vi "read_attributes.vi"(8 "error in (no error)":errorcluster, 11 "RadiusNeighborsRegressor in":refnum<class "RadiusNeighborsRegressor.lvclass">) -> (0 "error out":errorcluster, 2 "attributes":T1, 3 "RadiusNeighborsRegressor out":refnum<class "RadiusNeighborsRegressor.lvclass">)   [LabVIEW 2020, in "RadiusNeighborsRegressor.lvclass"]
uses:
  RadiusNeighborsRegressor.lvclass
  Controls/radius_neighbors_regressor_attributes.ctl
  RadiusNeighborsRegressor.lvclass/RadiusNeighborsRegressor.ctl
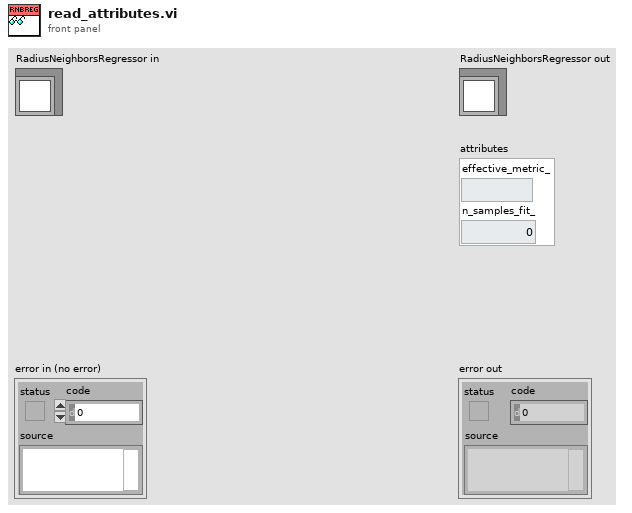
[diagram p1: front panel]
types:
  T1 = typedef "radius_neighbors_regressor_attributes.ctl" = cluster{"effective_metric_":string, "n_samples_fit_":dbl}
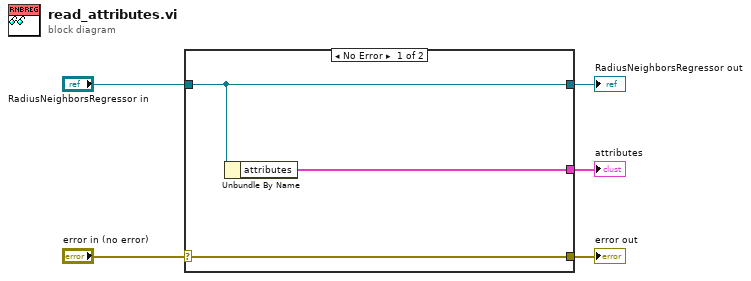
[diagram p0: block diagram]
diagram:
  n1 = case shown="No Error" "error in (no error)" {
    selector: "error in (no error)" -> [w8 w9]
    tunnel: [w8 w9] -> w4
    tunnel: [w7 w10] -> w2
    tunnel: "RadiusNeighborsRegressor in" -> [w7 w10]
    tunnel: [w6 _] -> w1
    frame No Error {
      n2 = Unbundle By Name(w7) -> ("attributes"=w6:T1)
    }
    frame Error {
    }
  }
  "error out" <- w4
  "RadiusNeighborsRegressor out" <- w2
  "attributes" <- w1
